vi "Get From Notification Map.vi"(7 "Alias":string, 8 "error in (no error)":errorcluster, 10 "Symbol Name":string, 11 "TwinCAT ADS in":refnum<class "TwinCAT ADS.lvclass">) -> (0 "error out":errorcluster, 2 "Value":T1={"Handle"=-1, "Cycle Time"=-1}, 3 "TwinCAT ADS out":refnum<class "TwinCAT ADS.lvclass">)   [LabVIEW 2018, in "TwinCAT ADS.lvclass"]
uses:
  TwinCAT ADS.lvclass
  Controls/Notifcation Map Value.ctl
  TwinCAT ADS.lvclass/TwinCAT ADS.ctl
  <vilib>/Utility/error.llb/Trim Whitespace.vi
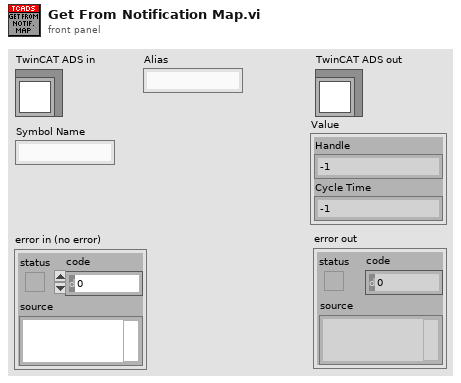
[diagram p1: front panel]
types:
  T1 = typedef "TwinCAT ADS.lvclass/Notifcation Map Value.ctl" = cluster{"Handle":i32, "Cycle Time":i32}
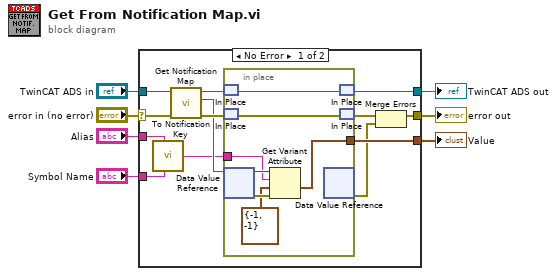
[diagram p0: block diagram]
diagram:
  n1 = case shown="No Error" "error in (no error)" {
    selector: "error in (no error)" -> [w12 w28]
    tunnel: "TwinCAT ADS in" -> [w18 w29]
    tunnel: "Symbol Name" -> [w15 _]
    tunnel: [w8 w28] -> w5
    tunnel: [w9 w29] -> w4
    tunnel: [w19 _] -> w2
    tunnel: "Alias" -> [w16 _]
    frame No Error {
      n2 = call "To Notification Key.vi"("Alias"=w16, "Symbol Name"=w15) -> ("Key"=w14:string)  [unwired: 5 in]
      n3 = call "Get Notification Map.vi"("error in (no error)"=w12, "TwinCAT ADS in"=w18) -> ("error out"=w20:errorcluster, "Notification Map"=w17:refnum<data-value>, "TwinCAT ADS out"=w13:refnum<class "TwinCAT ADS.lvclass">)  [unwired: 7 in]
      n4 = in-place {
        in-place-border: w14 -> [w24]
        in-place-border: [w27] -> w19
        n5 = in-place-match #1(w13) -> (w22:refnum<class "TwinCAT ADS.lvclass">)
        n6 = in-place-match #2(w20) -> (w21:errorcluster)
        n7 = in-place-dvr #3(w17) -> (w25:variant, w26:errorcluster)
        n8 = Get Variant Attribute(Variant=w25, name=w24, default value (empty Variant)=T1 {"Handle"=-1, "Cycle Time"=-1} ("Value"), error in=w26) -> (value=w27:T1)  [unwired: 3 out]
        n9 = in-place-dvr #3() -> (w10:errorcluster)  [unwired: 1 in, 1 out]
        n10 = in-place-match #1(w22) -> (w9:refnum<class "TwinCAT ADS.lvclass">)
        n11 = in-place-match #2(w21) -> (w11:errorcluster)
      }
      n12 = Merge Errors(w11, w10) -> (w8:errorcluster)
    }
    frame Error {
    }
  }
  "error out" <- w5
  "TwinCAT ADS out" <- w4
  "Value" <- w2
